vi "Follow Me Robot and Obstacle Avoidance.vi"() -> ()   [LabVIEW 2014]
doc: "This example shows how to track a green tennis ball with an AXIS M1011 camera, then control a Starter Kit robot to follow the ball.\n\nIt is strongly recommended that you configure the camera to acquire images at 320x240 resolution before running this example."
uses:
  <vilib>/myRIO/Instrument Drivers/Onboard IO/DIO/typedefs/DIO Reference.ctl
  <vilib>/myRIO/Common/Instrument Driver Framework/Utilities/typedefs/myRIO Generic Hardware Reference.ctl
  <vilib>/myRIO/Common/Instrument Driver Framework/Utilities/typedefs/Hardware Version Enum.ctl
  <vilib>/myRIO/Common/Instrument Driver Framework/Utilities/typedefs/myRIO v1.0 Reference.ctl
  <vilib>/myRIO/Common/Instrument Driver Framework/Utilities/typedefs/Generic FPGA Reference.ctl
  <vilib>/myRIO/Common/Instrument Driver Framework/myRIO v1.0/DIO/typedefs/DIO Channels List.ctl
  <vilib>/myRIO/Common/Instrument Driver Framework/myRIO v1.0/DIO/typedefs/DIO Channels Enum.ctl
  <vilib>/userdefined/High Color/nirio_resource_hc.ctl
  <vilib>/myRIO/Common/Instrument Driver Framework/Utilities/vis/Is FPGA Ref Available.vi
  <vilib>/myRIO/Common/Instrument Driver Framework/myRIO v1.0/DIO/vis/myRIO v1.1 Open DIO.vi
  <vilib>/myRIO/Instrument Drivers/Onboard IO/DIO/vis/Write.vi
  <vilib>/myRIO/Common/Instrument Driver Framework/Utilities/vis/Validate Channels.vi
  <vilib>/myRIO/Common/Instrument Driver Framework/myRIO v1.0/DIO/vis/myRIO v1.0 Reserve DIO.vi
  <vilib>/myRIO/Common/Instrument Driver Framework/myRIO v1.0/UART/vis/myRIO v1.0 Close UART.vi
  <vilib>/myRIO/Common/Instrument Driver Framework/myRIO v1.0/Resource Manager/vis/myRIO v1.0 Reserve Channel List.vi
  <vilib>/myRIO/Common/Instrument Driver Framework/myRIO v1.0/DIO/vis/myRIO v1.0 Build MUX Configuration DIO.vi
  <vilib>/myRIO/Common/Instrument Driver Framework/myRIO v1.0/Resource Manager/vis/myRIO v1.0 Reserve Channel.vi
  <vilib>/myRIO/Common/Instrument Driver Framework/myRIO v1.0/Resource Manager/vis/myRIO v1.0 Unreserve Channel.vi
  <vilib>/myRIO/Common/Instrument Driver Framework/myRIO v1.0/Resource Manager/vis/myRIO v1.0 Create Configuration List.vi
  <vilib>/myRIO/Common/Instrument Driver Framework/myRIO v1.0/Resource Manager/vis/myRIO v1.0 Build Mutex Name.vi
  <vilib>/Utility/VariantDataType/GetNumericInfo.vi
  <vilib>/Utility/error.llb/Error Cluster From Error Code.vi
  <vilib>/myRIO/Common/Instrument Driver Framework/myRIO v1.0/myRIO v1.1 Open.vi
  <vilib>/myRIO/Common/Instrument Driver Framework/Utilities/vis/IO Manager.vi
  <vilib>/myRIO/Common/Instrument Driver Framework/Utilities/vis/Configuration Manager.vi
  <vilib>/myRIO/Common/Instrument Driver Framework/myRIO v1.0/Resource Manager/vis/myRIO v1.0 Configure IO.vi
  <vilib>/myRIO/Common/Instrument Driver Framework/myRIO v1.0/myRIO v1.0 Close.vi
  <vilib>/myRIO/Common/Instrument Driver Framework/myRIO v1.0/DIO/vis/myRIO v1.0 Write DIO.vi
  <vilib>/myRIO/Common/Instrument Driver Framework/Utilities/vis/FPGA Ref Manager.vi
  <vilib>/myRIO/Common/Instrument Driver Framework/myRIO v1.0/myRIO v1.0 Reset FPGA.vi
  <vilib>/myRIO/Common/Instrument Driver Framework/myRIO v1.0/IRQ/vis/myRIO v1.0 IRQ Info FGV.vi
  <vilib>/myRIO/Common/Instrument Driver Framework/myRIO v1.0/IRQ/vis/myRIO v1.0 Timer IRQ Info FGV.vi
  <vilib>/myRIO/Common/Instrument Driver Framework/myRIO v1.0/IRQ/vis/myRIO v1.0 ISR Agent.vi
  <vilib>/myRIO/Express VI/Onboard Devices/LED/LED Express VI.xnode
  <vilib>/myRIO/Instrument Drivers/Onboard IO/DIO/vis/myRIO DIO Open.xnode
  TaimiOmni/vi.lib/robotics/TaimiOmni/TaimiOmni (RT)/TaimiOmni (RT).lvclass
  <vilib>/myRIO/Instrument Drivers/Utilities/Utilities.lvlib
  <vilib>/myRIO/Instrument Drivers/Onboard IO/DIO/DIO.lvlib
panel:
  out "IR2":dbl
  out "IR1":dbl
  out "XY Graph 2":cluster{"X":dbl, "Y":dbl}[](graph)
  out "RGB Image":T1(plugin-control)
  out "Forward Velocity (m/s)":dbl(slide) scale=-0.5..0.5
  out "Image":T1(plugin-control)
  in  "stop":bool
  out "CCW Velocity (rad/s)":dbl(slide) scale=2.0..-2.0
  out "Ball Found?":bool
  # "This example shows how to track a green tennis ball with an AXIS M1011 camera, then control a Starter Kit robot to follow the ball.\n\nIt is strongly recommended that you configure the camera to acquire images at 320x240 resolution before running this example."
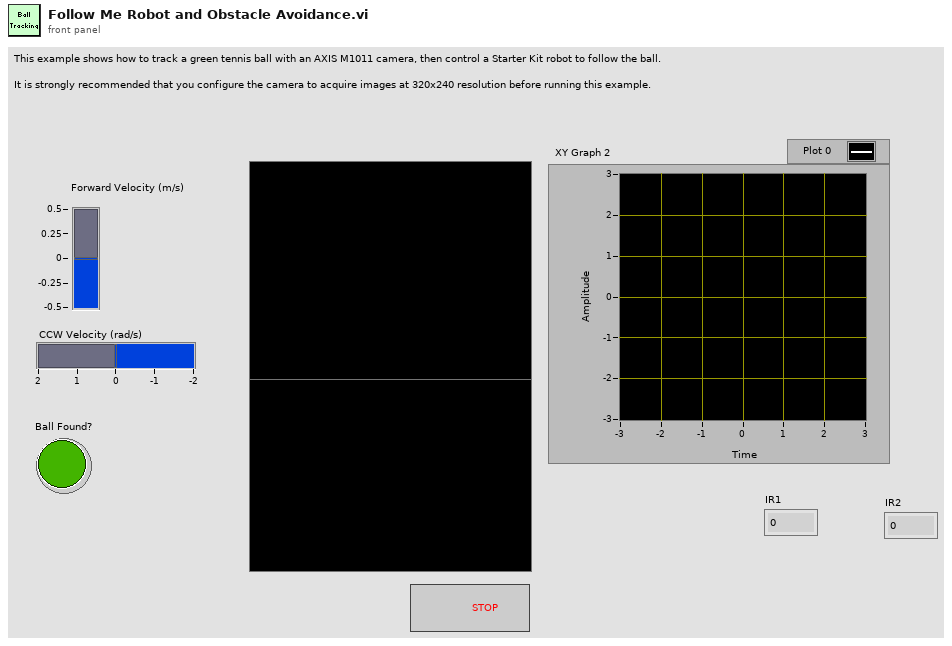
[diagram p1: front panel]
types:
  T1 = typedef "IMAQ Image.ctl" = refnum<image>
  T2 = typedef "Ball Tracking Image Refs.ctl" = cluster{"acquired image":T1, "threshold image":T1, "Video Handle out":i64, "Kinect Handle":i64, "Video and Depth config":cluster{"Video Resolution":T3, "Video Format":T4, "Depth Format":T5, "Depth Resolution":T6}}
  T3 = typedef "Video Resolution Control.ctl" = enum32{"FREENECT_RESOLUTION_LOW", "FREENECT_RESOLUTION_MEDIUM", "FREENECT_RESOLUTION_HIGH"}
  T4 = typedef "Video Format Control.ctl" = enum32{"FREENECT_VIDEO_RGB", "FREENECT_VIDEO_BAYER", "FREENECT_VIDEO_IR_8BIT", "FREENECT_VIDEO_IR_10BIT", "FREENECT_VIDEO_IR_10BIT_PACKED", "FREENECT_VIDEO_YUV_RGB", "FREENECT_VIDEO_YUV_RAW"}
  T5 = typedef "Depth Format Control.ctl" = enum32{"FREENECT_DEPTH_11BIT", "FREENECT_DEPTH_10BIT", "FREENECT_DEPTH_11BIT_PACKED", "FREENECT_DEPTH_10BIT_PACKED", "FREENECT_DEPTH_REGISTERED", "FREENECT_DEPTH_MM"}
  T6 = typedef "Depth Resolution Control.ctl" = enum16{"FREENECT_RESOLUTION_TINY", "FREENECT_RESOLUTION_LOW", "FREENECT_RESOLUTION_MEDIUM"}
  T7 = typedef "DIO.lvlib/DIO Reference.ctl" = cluster{"myRIO Reference":T8, "DIO Channels List":T12}
  T8 = typedef "myRIO Generic Hardware Reference.ctl" = cluster{"myRIO Model":T9, "myRIO Hardware Reference":T10}
  T9 = typedef "Hardware Version Enum.ctl" = enum16{"Unknown", "myRIO-1900", "myRIO-1950"}
  T10 = typedef "myRIO v1.0 Reference.ctl" = cluster{"Generic FPGA Reference":T11, "Allow multiple opens":bool}
  T11 = typedef "Generic FPGA Reference.ctl" = refnum<k20>
  T12 = typedef "DIO Channels List.ctl" = T13[]
  T13 = typedef "DIO Channels Enum.ctl" = enum16{"Not Connected", "C/DIO0", "C/DIO1", "C/DIO2", "C/DIO3", "C/DIO4", "C/DIO5", "C/DIO6", "C/DIO7", "A/DIO0", "A/DIO1", "A/DIO2", "A/DIO3", "A/DIO4", "A/DIO5", "A/DIO6", "A/DIO7", "A/DIO8", "A/DIO9", "A/DIO10", "A/DIO11", "A/DIO12", "A/DIO13", "A/DIO14", "A/DIO15", "B/DIO0", "B/DIO1", "B/DIO2", "B/DIO3", "B/DIO4", "B/DIO5", "B/DIO6", "B/DIO7", "B/DIO8", "B/DIO9", "B/DIO10", "B/DIO11", "B/DIO12", "B/DIO13", "B/DIO14", "B/DIO15", "LED0", "LED1", "LED2", "LED3", "Button0"}
  T14 = typedef "nirio_resource_hc.ctl" = tag
  T15 = typedef "Ball Pixel Info.ctl" = cluster{"x position":dbl, "y position":dbl, "area":dbl}
  T16 = typedef "TaimiOmni.lvclass/TaimiOmniIRData.ctl" = cluster{"distance":dbl, "angle":dbl}
  T17 = cluster{"steering frame velocity[0]":dbl, "steering frame velocity[1]":dbl, "steering frame velocity[2]":dbl}
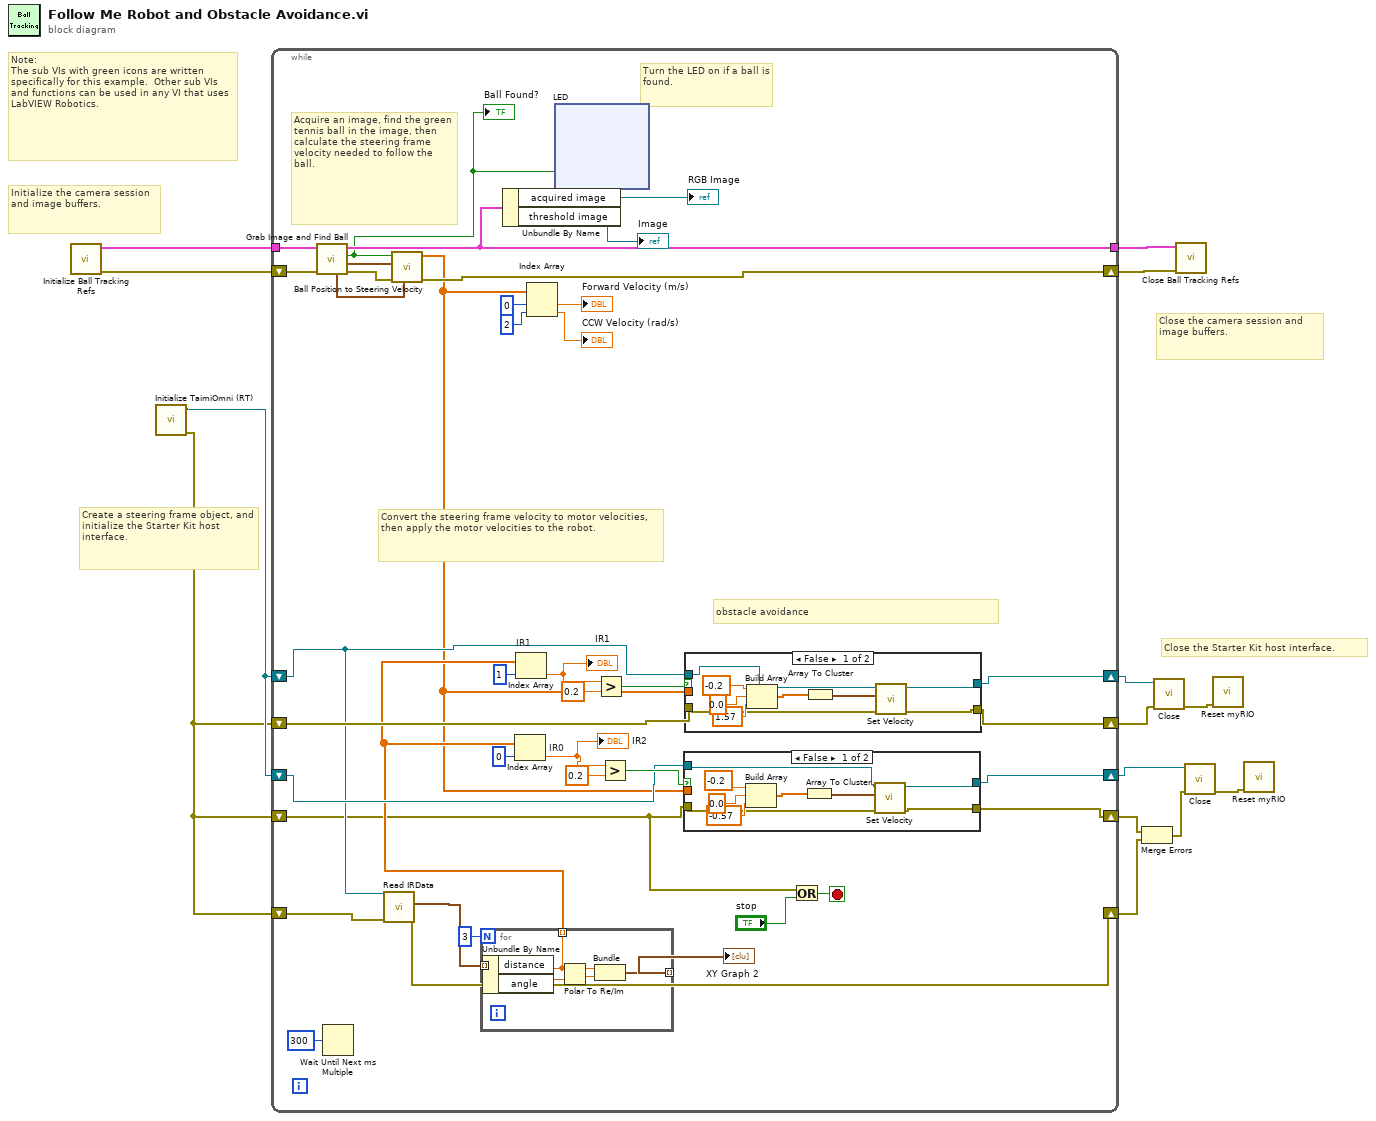
[diagram p0: block diagram]
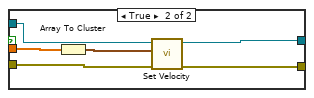
[diagram p2: hidden frame]
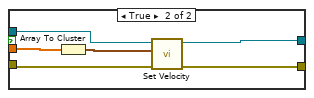
[diagram p3: hidden frame]
diagram:
  # "Note:\nThe sub VIs with green icons are written specifically for this example.  Other sub VIs and functions can be used in any VI that uses LabVIEW Robotics."
  # "Close the Starter Kit host interface."
  # "Close the camera session and image buffers."
  # "Create a steering frame object, and initialize the Starter Kit host interface."
  # "Initialize the camera session and image buffers."
  n1 = call "Initialize Ball Tracking Refs.vi"() -> ("error out"=w11:errorcluster, "ball tracking refs"=w14:T2)  [unwired: 10 in]
  n2 = call "Initialize TaimiOmni (RT).vi"() -> ("error out"=w5:errorcluster, "TaimiOmni (RT) out"=w8:refnum<class "TaimiOmni (RT).lvclass">)  [unwired: 10 in]
  n3 = while {
    shift-right: [w40] -> w12
    shift-left: w11 -> [w54]
    tunnel: w14 -> [w51]
    tunnel: [w50] -> w13
    shift-right: [w32] -> w9
    shift-left: w8 -> [w17]
    shift-right: [w31] -> w6
    shift-left: w8 -> [w30]
    shift-right: [w28] -> w3
    shift-left: w5 -> [w29]
    shift-right: [w26] -> w4
    shift-left: w5 -> [w27]
    shift-right: [w25] -> w2
    shift-left: w5 -> [w16]
    stop <- w52 stop-if-true
    # "obstacle avoidance"
    # "Convert the steering frame velocity to motor velocities, then apply the motor velocities to the robot."
    # "Acquire an image, find the green tennis ball in the image, then calculate the steering frame velocity needed to follow the ball."
    # "Turn the LED on if a ball is found."
    n4 = call "Grab Image and Find Ball.vi"("error in (no error)"=w54, "ball tracking refs in"=w51) -> ("error out"=w45:errorcluster, "ball pixel position"=w46:T15, "ball found?"=w39:bool, "ball tracking refs out"=w50:T2, "image resolution"=w43:cluster{"x":i32, "y":i32})  [unwired: 5 in]
    "Ball Found?" <- w39
    n5 = Wait Until Next ms Multiple(millisecond multiple=u32 300 ("milliseconds to wait")) -> ()  [unwired: 1 out]
    n6 = call-dynamic "Read IRData.vi"("error in (no error)"=w29, "TaimiOmni in"=w17) -> ("error out"=w28:errorcluster, "IRData"=w22:T16[])  [unwired: 7 in, 1 out]
    n7 = call "Ball Position to Steering Velocity.vi"("image resolution"=w43, "error in (no error)"=w45, "ball pixel position"=w46, "ball found?"=w39) -> ("error out"=w40:errorcluster, "steering frame velocity"=w15:dbl[])  [unwired: 6 in]
    n8 = for {
      N: 3 -> [_]
      tunnel: w22 -> [w90] mode=indexing
      tunnel: [w87] -> w37 mode=indexing
      tunnel: [w85] -> w21 mode=indexing
      n9 = Unbundle By Name(w90) -> ("distance"=w85:dbl, "angle"=w86:dbl)
      n10 = Polar To Re/Im(2:w86, 3:w85) -> (0:w88:dbl, 1:w89:dbl)
      n11 = Bundle(w89, w88) -> (w87:cluster{dbl, dbl})  [unwired: 1 in]
    }
    "XY Graph 2" <- w37
    n12 = Unbundle By Name(w50) -> ("acquired image"=→"RGB Image":T1, "threshold image"=→"Image":T1)
    n13 = Index Array "IR0"(array=w21, index=0) -> (element=w23:dbl)
    "IR2" <- w23
    n14 = Index Array "IR1"(array=w21, index=1) -> (element=w24:dbl)
    "IR1" <- w24
    n15 = Index Array(array=w15, index #1=0 ("index"), index #2=2 ("index")) -> (element #1=→"Forward Velocity (m/s)":dbl, element #2=→"CCW Velocity (rad/s)":dbl)
    n16 = xnode "LED"("LED0"=w39) -> ()  [unwired: 1 in, 1 out]
    n17 = Greater?(x=w24, y=0.2) -> (0:w35:bool)
    n18 = Greater?(x=w23, y=0.2) -> (0:w33:bool)
    n19 = case shown="False" w33 {
      tunnel: w15 -> [_ w69]
      tunnel: [w61 w67] -> w31
      tunnel: w16 -> [w56 w66]
      tunnel: w30 -> [w57 w65]
      tunnel: [w55 w64] -> w25
      frame False {
        n20 = Build Array(-0.2, 0.0, -0.57 ("element")) -> (w59:dbl[])
        n21 = Array To Cluster(array=w59) -> (cluster=w60:cluster{"[0]":dbl, "[1]":dbl, "[2]":dbl})
        n22 = call-dynamic "Set Velocity.vi"("error in (no error)"=w56, "TaimiOmniVelocity"=w60, "TaimiOmni in"=w57) -> ("error out"=w55:errorcluster, "TaimiOmni out"=w61:refnum<class "TaimiOmni (RT).lvclass">)  [unwired: 7 in]
      }
      frame True {
        n23 = Array To Cluster(array=w69) -> (cluster=w68:T17)
        n24 = call-dynamic "Set Velocity.vi"("error in (no error)"=w66, "TaimiOmniVelocity"=w68, "TaimiOmni in"=w65) -> ("error out"=w64:errorcluster, "TaimiOmni out"=w67:refnum<class "TaimiOmni (RT).lvclass">)  [unwired: 7 in]
      }
    }
    n25 = case shown="False" w35 {
      tunnel: w15 -> [_ w84]
      tunnel: [w77 w82] -> w32
      tunnel: w27 -> [w72 w81]
      tunnel: [w71 w80] -> w26
      tunnel: w17 -> [w73 w79]
      frame False {
        n26 = Build Array(-0.2, 0.0, 1.57 ("element")) -> (w75:dbl[])
        n27 = Array To Cluster(array=w75) -> (cluster=w76:cluster{"[0]":dbl, "[1]":dbl, "[2]":dbl})
        n28 = call-dynamic "Set Velocity.vi"("error in (no error)"=w72, "TaimiOmniVelocity"=w76, "TaimiOmni in"=w73) -> ("error out"=w71:errorcluster, "TaimiOmni out"=w77:refnum<class "TaimiOmni (RT).lvclass">)  [unwired: 7 in]
      }
      frame True {
        n29 = Array To Cluster(array=w84) -> (cluster=w83:T17)
        n30 = call-dynamic "Set Velocity.vi"("error in (no error)"=w81, "TaimiOmniVelocity"=w83, "TaimiOmni in"=w79) -> ("error out"=w80:errorcluster, "TaimiOmni out"=w82:refnum<class "TaimiOmni (RT).lvclass">)  [unwired: 7 in]
      }
    }
    n31 = Or(x=w16, y="stop") -> (x .or. y?=w52:bool)
  }
  n32 = Merge Errors(w2, w3) -> (w1:errorcluster)
  n33 = call-dynamic "Close.vi"("error in (no error)"=w4, "TaimiOmni in"=w9) -> ("error out"=w10:errorcluster)  [unwired: 9 in]
  n34 = call "Close Ball Tracking Refs.vi"("error in (no error)"=w12, "ball tracking refs"=w13) -> ()  [unwired: 9 in, 1 out]
  n35 = call-dynamic "Close.vi"("error in (no error)"=w1, "TaimiOmni in"=w6) -> ("error out"=w7:errorcluster)  [unwired: 9 in]
  n36 = call <vilib>:"Reset myRIO.vi"("error in (no error)"=w10) -> ()  [unwired: 10 in, 1 out]
  n37 = call <vilib>:"Reset myRIO.vi"("error in (no error)"=w7) -> ()  [unwired: 10 in, 1 out]
